vi "Main.vi"() -> ()   [LabVIEW 2020, in "Game.lvclass"]
uses:
  Game.lvclass
  Particle/Position.ctl
  Snake/Direction.ctl
  Particle.lvclass
  C:/git/astemes-snake-game/source/Drawable/Drawable.lvclass
  Snake/Snake.lvclass
  World/World.lvclass
  Game Board/Game Board.lvclass
panel:
  in  "Right":bool
  in  "Left":bool
  in  "Down":bool
  in  "Up":bool
  in  "stop":bool
  out "game Board":u32[][](array[colorbox])
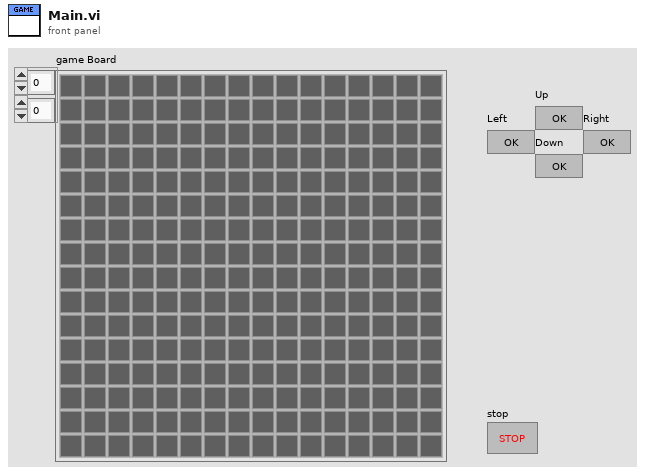
[diagram p1: front panel]
types:
  T1 = typedef "Particle.lvclass/Position.ctl" = cluster{"X":i32, "Y":i32}
  T2 = typedef "Snake.lvclass/Direction.ctl" = enum16{"X", "-X", "Y", "-Y"}
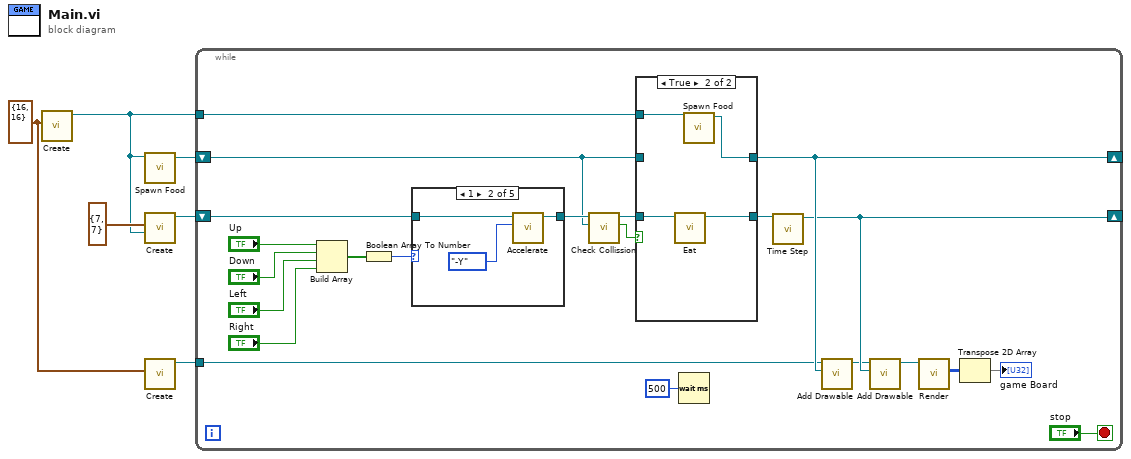
[diagram p0: block diagram]
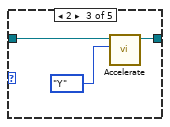
[diagram p3: hidden frame]
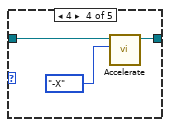
[diagram p4: hidden frame]
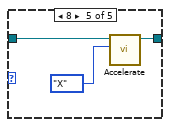
[diagram p5: hidden frame]
diagram:
  w1 = T1 {"X"=16, "Y"=16} ("Size")
  n1 = call "Create.vi"("Size"=w1) -> ("World out"=w3:refnum<class "World.lvclass">)  [unwired: 10 in]
  n2 = call "Spawn Food.vi"("World in"=w3) -> ("Particle out"=w4:refnum<class "Particle.lvclass">)  [unwired: 10 in]
  n3 = call "Create.vi"("World.lvclass"=w3, "Position"=T1 {"X"=7, "Y"=7}) -> ("Snake out"=w5:refnum<class "Snake.lvclass">)  [unwired: 9 in]
  n4 = call "Create.vi"("Size"=w1) -> ("Game Board out"=w2:refnum<class "Game Board.lvclass">)  [unwired: 10 in]
  n5 = while {
    shift-right: [w20] -> _
    shift-left: w5 -> [w28]
    shift-right: [w22] -> _
    shift-left: w4 -> [w24]
    tunnel: w3 -> [w23]
    tunnel: w2 -> [w17]
    stop <- "stop" stop-if-true
    n6 = Build Array("Up", "Down", "Left", "Right") -> (w8:bool[])
    n7 = Boolean Array To Number(Boolean array=w8) -> (number=w7:u32)
    n8 = case shown="1" w7 {
      tunnel: w28 -> [w29 w32 w35 w38 w41]
      tunnel: [w29 w31 w34 w37 w40] -> w27
      frame Default {
      }
      frame 1 {
        n9 = call "Accelerate.vi"("Direction"=Direction."-Y", "Snake in"=w32) -> ("Snake out"=w31:refnum<class "Snake.lvclass">)  [unwired: 9 in]
      }
      frame 2 {
        n10 = call "Accelerate.vi"("Direction"=Direction."Y", "Snake in"=w35) -> ("Snake out"=w34:refnum<class "Snake.lvclass">)  [unwired: 9 in]
      }
      frame 4 {
        n11 = call "Accelerate.vi"("Direction"=Direction."-X", "Snake in"=w38) -> ("Snake out"=w37:refnum<class "Snake.lvclass">)  [unwired: 9 in]
      }
      frame 8 {
        n12 = call "Accelerate.vi"("Direction"=Direction."X", "Snake in"=w41) -> ("Snake out"=w40:refnum<class "Snake.lvclass">)  [unwired: 9 in]
      }
    }
    n13 = call "Check Collission.vi"("Particle"=w24, "Snake in"=w27) -> ("Collided?"=w25:bool, "Snake out"=w26:refnum<class "Snake.lvclass">)  [unwired: 8 in]
    n14 = case shown="True" w25 {
      tunnel: w26 -> [w42 w47]
      tunnel: [w42 w46] -> w21
      tunnel: w24 -> [w43 _]
      tunnel: w23 -> [_ w45]
      tunnel: [w43 w44] -> w22
      frame False {
      }
      frame True {
        n15 = call "Eat.vi"("Snake in"=w47) -> ("Snake out"=w46:refnum<class "Snake.lvclass">)  [unwired: 10 in]
        n16 = call "Spawn Food.vi"("World in"=w45) -> ("Particle out"=w44:refnum<class "Particle.lvclass">)  [unwired: 10 in]
      }
    }
    n17 = Wait (ms)(milliseconds to wait=u32 500) -> ()  [unwired: 1 out]
    n18 = call "Time Step.vi"("Snake in"=w21) -> ("Snake out"=w20:refnum<class "Snake.lvclass">)  [unwired: 10 in]
    n19 = call "Add Drawable.vi"("Drawable"=w22, "Game Board in"=w17) -> ("Game Board out"=w19:refnum<class "Game Board.lvclass">)  [unwired: 9 in]
    n20 = call "Add Drawable.vi"("Drawable"=w20, "Game Board in"=w19) -> ("Game Board out"=w18:refnum<class "Game Board.lvclass">)  [unwired: 9 in]
    n21 = call "Render.vi"("Game Board in"=w18) -> ("game Board"=w16:u32[][])  [unwired: 9 in, 1 out]
    n22 = Transpose 2D Array(2D array=w16) -> (transposed array=→"game Board":u32[][])
  }
